vi "Is Point in Rectangular ROI.vi"(8 "error in (no error)":errorcluster, 9 "Y":dbl, 10 "X":dbl, 11 "ROI Contour":T1 {"Type" items=["No Selection", "Point", "Line", "Rectangle", "Oval", "Polygon", "Freehand Region", "Annulus", "Unused2", "Unused3", "Broken Line", "Freehand Line", "Rotated Rectangle"]}) -> (0 "error out":errorcluster, 3 "Is in ROI?":bool)   [LabVIEW 2021, in "Image.lvlib"]
uses:
  Image.lvlib
  ROI  Type.ctl
  <vilib>/Utility/error.llb/Error Cluster From Error Code.vi
  <vilib>/ErrorRing/Error Ring.xnode
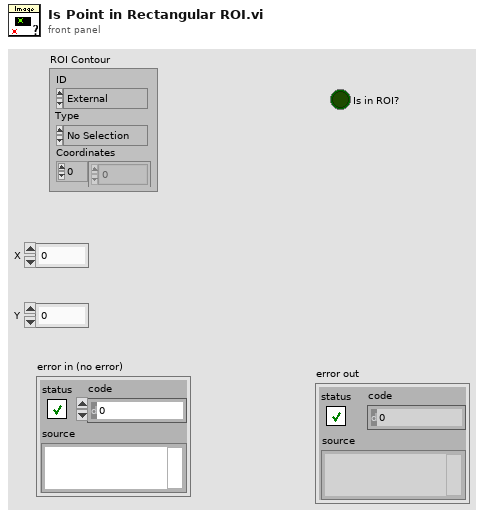
[diagram p1: front panel]
types:
  T1 = cluster{"ID":enum32{"External", "Internal"}, "Type":u32, "Coordinates":i32[]}
  T2 = typedef "Image.lvlib/ROI  Type.ctl" = enum16{"Point", "Oval", "Rectangle"}
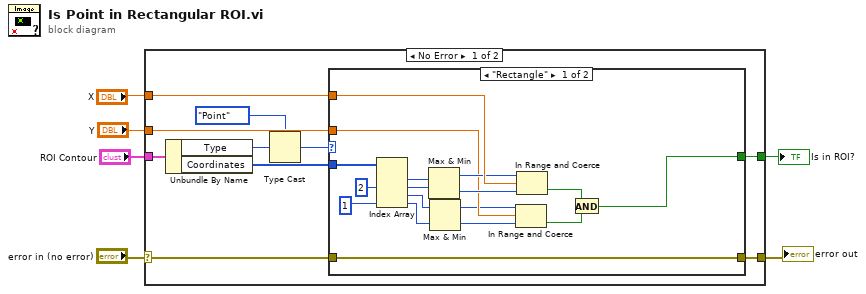
[diagram p0: block diagram]
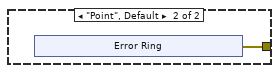
[diagram p2: hidden frame]
diagram:
  n1 = case shown="No Error" "error in (no error)" {
    selector: "error in (no error)" -> [w7 w39]
    tunnel: "ROI Contour" -> [w15 _]
    tunnel: "X" -> [w14 _]
    tunnel: "Y" -> [w13 _]
    tunnel: [w12 _] -> w1
    tunnel: [w8 w39] -> w2
    frame No Error {
      n2 = Unbundle By Name(w15) -> ("Type"=w11:u32, "Coordinates"=w16:i32[])
      n3 = Type Cast(type=ROI__Type."Point" ("Type"), x=w11) -> (*(type *) &x=w9:T2)
      n4 = case shown="\"Rectangle\"" w9 {
        tunnel: w16 -> [w32 _]
        tunnel: w14 -> [w31 _]
        tunnel: w13 -> [w22 _]
        tunnel: [w17 _] -> w12
        tunnel: [w33 w34] -> w8
        tunnel: w7 -> [w33 _]
        frame "Rectangle" {
          n5 = Index Array(array=w32, index #2=2 ("index"), index #4=1 ("index")) -> (element #1=w28:i32, element #2=w27:i32, element #3=w26:i32, element #4=w25:i32)  [unwired: 2 in]
          n6 = Max & Min(x=w28, y=w27) -> (max(x,y)=w24:i32, min(x,y)=w23:i32)
          n7 = Max & Min(x=w26, y=w25) -> (max(x,y)=w21:i32, min(x,y)=w20:i32)
          n8 = In Range and Coerce(upper limit=w21, x=w22, lower limit=w20) -> (In Range?=w18:bool)  [unwired: 1 out]
          n9 = In Range and Coerce(upper limit=w24, x=w31, lower limit=w23) -> (In Range?=w19:bool)  [unwired: 1 out]
          n10 = And(x=w19, y=w18) -> (x .and. y?=w17:bool)
        }
        frame "Point", Default {
          n11 = xnode "Error Ring"() -> ("error out"=w34:errorcluster)
        }
      }
    }
    frame Error {
    }
  }
  "error out" <- w2
  "Is in ROI?" <- w1
